vi "Read INI File (PV).vi"(8 "error in":errorcluster, 11 "Path":path) -> (0 "error out":errorcluster, 1 "Scaling Coefficients":T1, 2 "DER_Info":T4)   [LabVIEW 2018]
uses:
  <vilib>/ORNL/CSEISMIC DDS/CSEISMIC DDS Base/Data Types/DER_Info.ctl
  <vilib>/ORNL/CSEISMIC DDS/CSEISMIC DDS Base/Data Types/Controls/DeviceID.ctl
  Controls/Scaling Coefficients Cluster.ctl
  Controls/Scaling Coefficients Measurements.ctl
  Controls/Scaling Coefficients Setpoints.ctl
  <vilib>/Utility/config.llb/NI_LVConfig.lvlib
  <vilib>/ORNL/CSEISMIC DDS/CSEISMIC DDS Base/CSEISMIC DDS.lvclass
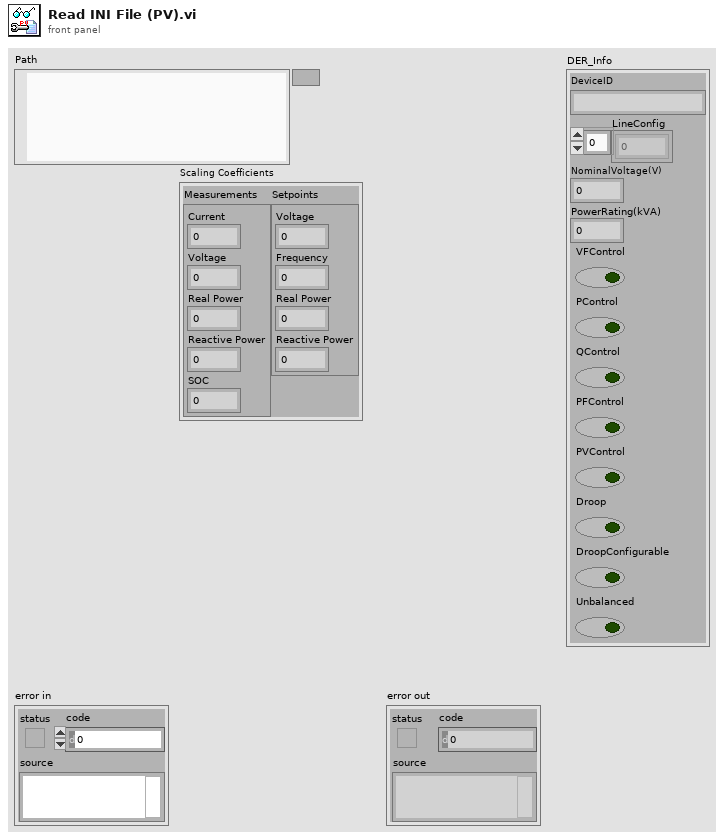
[diagram p1: front panel]
types:
  T1 = typedef "Scaling Coefficients Cluster.ctl" = cluster{"Measurements":T2, "Setpoints":T3}
  T2 = typedef "Scaling Coefficients Measurements.ctl" = cluster{"Current":dbl, "Voltage":dbl, "Real Power":dbl, "Reactive Power":dbl, "SOC":dbl}
  T3 = typedef "Scaling Coefficients Setpoints.ctl" = cluster{"Voltage":dbl, "Frequency":dbl, "Real Power":dbl, "Reactive Power":dbl}
  T4 = typedef "CSEISMIC DDS.lvlib/CSEISMIC DDS.lvclass/DER_Info.ctl" = cluster{"DeviceID":T5, "LineConfig":u8[], "NominalVoltage(V)":dbl, "PowerRating(kVA)":dbl, "VFControl":bool, "PControl":bool, "QControl":bool, "PFControl":bool, "PVControl":bool, "Droop":bool, "DroopConfigurable":bool, "Unbalanced":bool}
  T5 = typedef "CSEISMIC DDS.lvlib/CSEISMIC DDS.lvclass/DeviceID.ctl" = string
  T6 = typedef "NI_LVConfig.lvlib/Config Data RefNum.ctl" = refnum<k1>
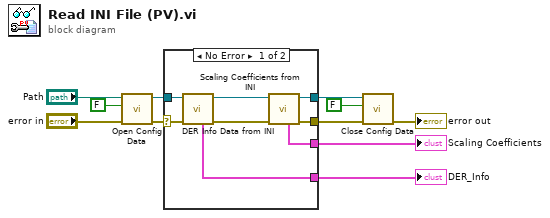
[diagram p0: block diagram]
diagram:
  n1 = call <vilib>:"Open Config Data.vi"("error in (no error)"="error in", "create file if necessary (T)"=FALSE, "configuration file path"="Path") -> ("error out"=w9:errorcluster, "refnum"=w8:T6)  [unwired: 6 in, 1 out]
  n2 = case shown="No Error" w9 {
    selector: w9 -> [w18 w20]
    tunnel: w8 -> [w19 w21]
    tunnel: [w17 _] -> w4
    tunnel: [w16 w21] -> w7
    tunnel: [w15 w20] -> w6
    tunnel: [w14 _] -> w1
    frame No Error {
      n3 = call "DER Info Data from INI.vi"("error in"=w18, "Config Refnum in"=w19) -> ("error out"=w12:errorcluster, "Config Refnum out"=w13:T6, "DER_Info"=w17:T4)  [unwired: 7 in]
      n4 = call "Scaling Coefficients from INI.vi"("error in"=w12, "Config Refnum in"=w13) -> ("error out"=w15:errorcluster, "Config Refnum out"=w16:T6, "Scaling Coefficients"=w14:T1)  [unwired: 7 in]
    }
    frame Error {
    }
  }
  "DER_Info" <- w4
  "Scaling Coefficients" <- w1
  n5 = call <vilib>:"Close Config Data.vi"("error in (no error)"=w6, "write file if changed (T)"=FALSE, "refnum"=w7) -> ("error out"=→"error out":errorcluster)  [unwired: 7 in, 1 out]
